vi "Build BC Schedule.vi"(8 "error in (no error)":errorcluster, 11 "Bus Controller in":refnum<class "Bus Controller.lvclass">) -> (0 "error out":errorcluster, 3 "Bus Controller out":refnum<class "Bus Controller.lvclass">)   [LabVIEW 2020, in "Unit Tests.lvlib" / "Bus Controller.lvclass"]
uses:
  Bus Controller.lvclass
  Bus Controller/TypeDefs/Bus Controller Configuration.ctl
  Bus Controller/TypeDefs/Bus Controller Timeout.ctl
  Frames & Messages/TypeDefs/RT-RT Message Config.ctl
  Frames & Messages/TypeDefs/Command Config.ctl
  Frames & Messages/TypeDefs/Command Type.ctl
  Frames & Messages/TypeDefs/Command Terminal Address.ctl
  Frames & Messages/TypeDefs/Command SubAddress.ctl
  Frames & Messages/TypeDefs/Command Word Count.ctl
  Frames & Messages/TypeDefs/Message Config.ctl
  Frames & Messages/TypeDefs/Message Control.ctl
  Frames & Messages/TypeDefs/Simplified Parameter Data Table.ctl
  Frames & Messages/TypeDefs/Scaling Information.ctl
  Bus Controller.lvclass/Bus Controller.ctl
  Frames & Messages/RT-RT Message/RT-RT Message.lvclass
  C:/Users/MattJ/Desktop/git/bci-1553-labview-api/src/Frames & Messages/Message/Message.lvclass
  Bus Controller/Bus Controller.lvclass
  C:/Users/MattJ/Desktop/git/bci-1553-labview-api/src/1553 SubComponent/1553 SubComponent.lvclass
  Frames & Messages/Major Frame/Major Frame.lvclass
  1553 Session/1553 Session.lvclass
  BCI-1553 API.lvlib
  Frames & Messages/Message/Message.lvclass
  Frames & Messages/Minor Frame/Minor Frame.lvclass
  1553 Component/1553 Component.lvclass
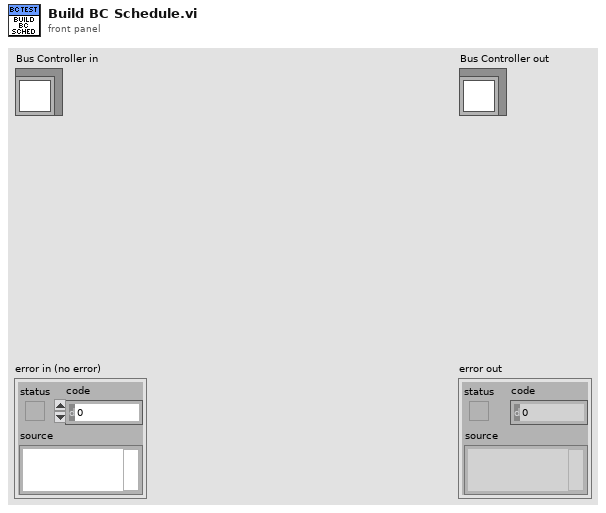
[diagram p1: front panel]
types:
  T1 = typedef "BCI-1553 API.lvlib/Command Type.ctl" = enum16{"Transmit", "Receive"}
  T2 = typedef "BCI-1553 API.lvlib/Command Terminal Address.ctl" = enum16{"0", "1", "2", "3", "4", "5", "6", "7", "8", "9", "10", "11", "12", "13", "14", "15", "16", "17", "18", "19", "20", "21", "22", "23", "24", "25", "26", "27", "28", "29", "30", "Broadcast"}
  T3 = typedef "BCI-1553 API.lvlib/Command SubAddress.ctl" = enum16{"Mode Code", "1", "2", "3", "4", "5", "6", "7", "8", "9", "10", "11", "12", "13", "14", "15", "16", "17", "18", "19", "20", "21", "22", "23", "24", "25", "26", "27", "28", "29", "30"}
  T4 = typedef "BCI-1553 API.lvlib/Command Word Count.ctl" = enum16{"1", "2", "3", "4", "5", "6", "7", "8", "9", "10", "11", "12", "13", "14", "15", "16", "17", "18", "19", "20", "21", "22", "23", "24", "25", "26", "27", "28", "29", "30", "31", "32"}
  T5 = typedef "BCI-1553 API.lvlib/Message Config.ctl" = cluster{"Time to Next Msg (4 us)":u16, "Command Config":T6, "Message Control":T7}
  T6 = typedef "BCI-1553 API.lvlib/Command Config.ctl" = cluster{"Command Type":T1, "Terminal Address":T2, "SubAddress":T3, "Word Count\\Mode Code":T4, "Command Data":u16[]}
  T7 = typedef "BCI-1553 API.lvlib/Message Control.ctl" = cluster{"MC17 Time Sync":bool, "Error Mask":bool, "Service Request Mask":bool, "Busy Mask":bool, "SubSystem Flag Mask":bool, "Terminal Flag Mask":bool, "Reserved Mask":bool, "Retry":bool, "Bus A / !Bus B":bool, "Self-Test Loopback":bool, "Broadcast Mask":bool, "EoM Interrupt":bool, "Mode Code Format":bool, "Broadcast Format":bool, "RT-RT Format":bool}
  T8 = typedef "BCI-1553 API.lvlib/RT-RT Message Config.ctl" = cluster{"Tx Command Config":T6}
  T9 = typedef "BCI-1553 API.lvlib/Bus Controller.lvclass/Bus Controller Configuration.ctl" = cluster{"Timeout":T10, "BC Retry":bool, "BC Second Retry":bool, "BC Retry Alt Bus":bool, "BC Second Retry Alt Bus":bool, "BC Retry on Status Bit":bool, "Msg Error No Data Valid":bool, "Busy Status No Data Valid":bool, "Msg Gap Timer":bool, "Watchdog Timer":bool, "Time Tag Sync":bool, "Even Time Tag Sync":bool, "Gap Check":bool, "Broadcast Mask Enable":bool}
  T10 = typedef "BCI-1553 API.lvlib/Bus Controller.lvclass/Bus Controller Timeout.ctl" = enum16{"17us", "22us", "60us", "140us"}
  T11 = typedef "BCI-1553 API.lvlib/Simplified Parameter Data Table.ctl" = cluster{"Parameter Name":string, "Base Word":u16, "Scaling Info":T12}
  T12 = typedef "BCI-1553 API.lvlib/Scaling Information.ctl" = cluster{"Bit Offset":i32, "Bit Count":i32, "LSB Resolution":dbl, "2's Complement":bool, "Big Endian":bool, "Sign Bit":bool}
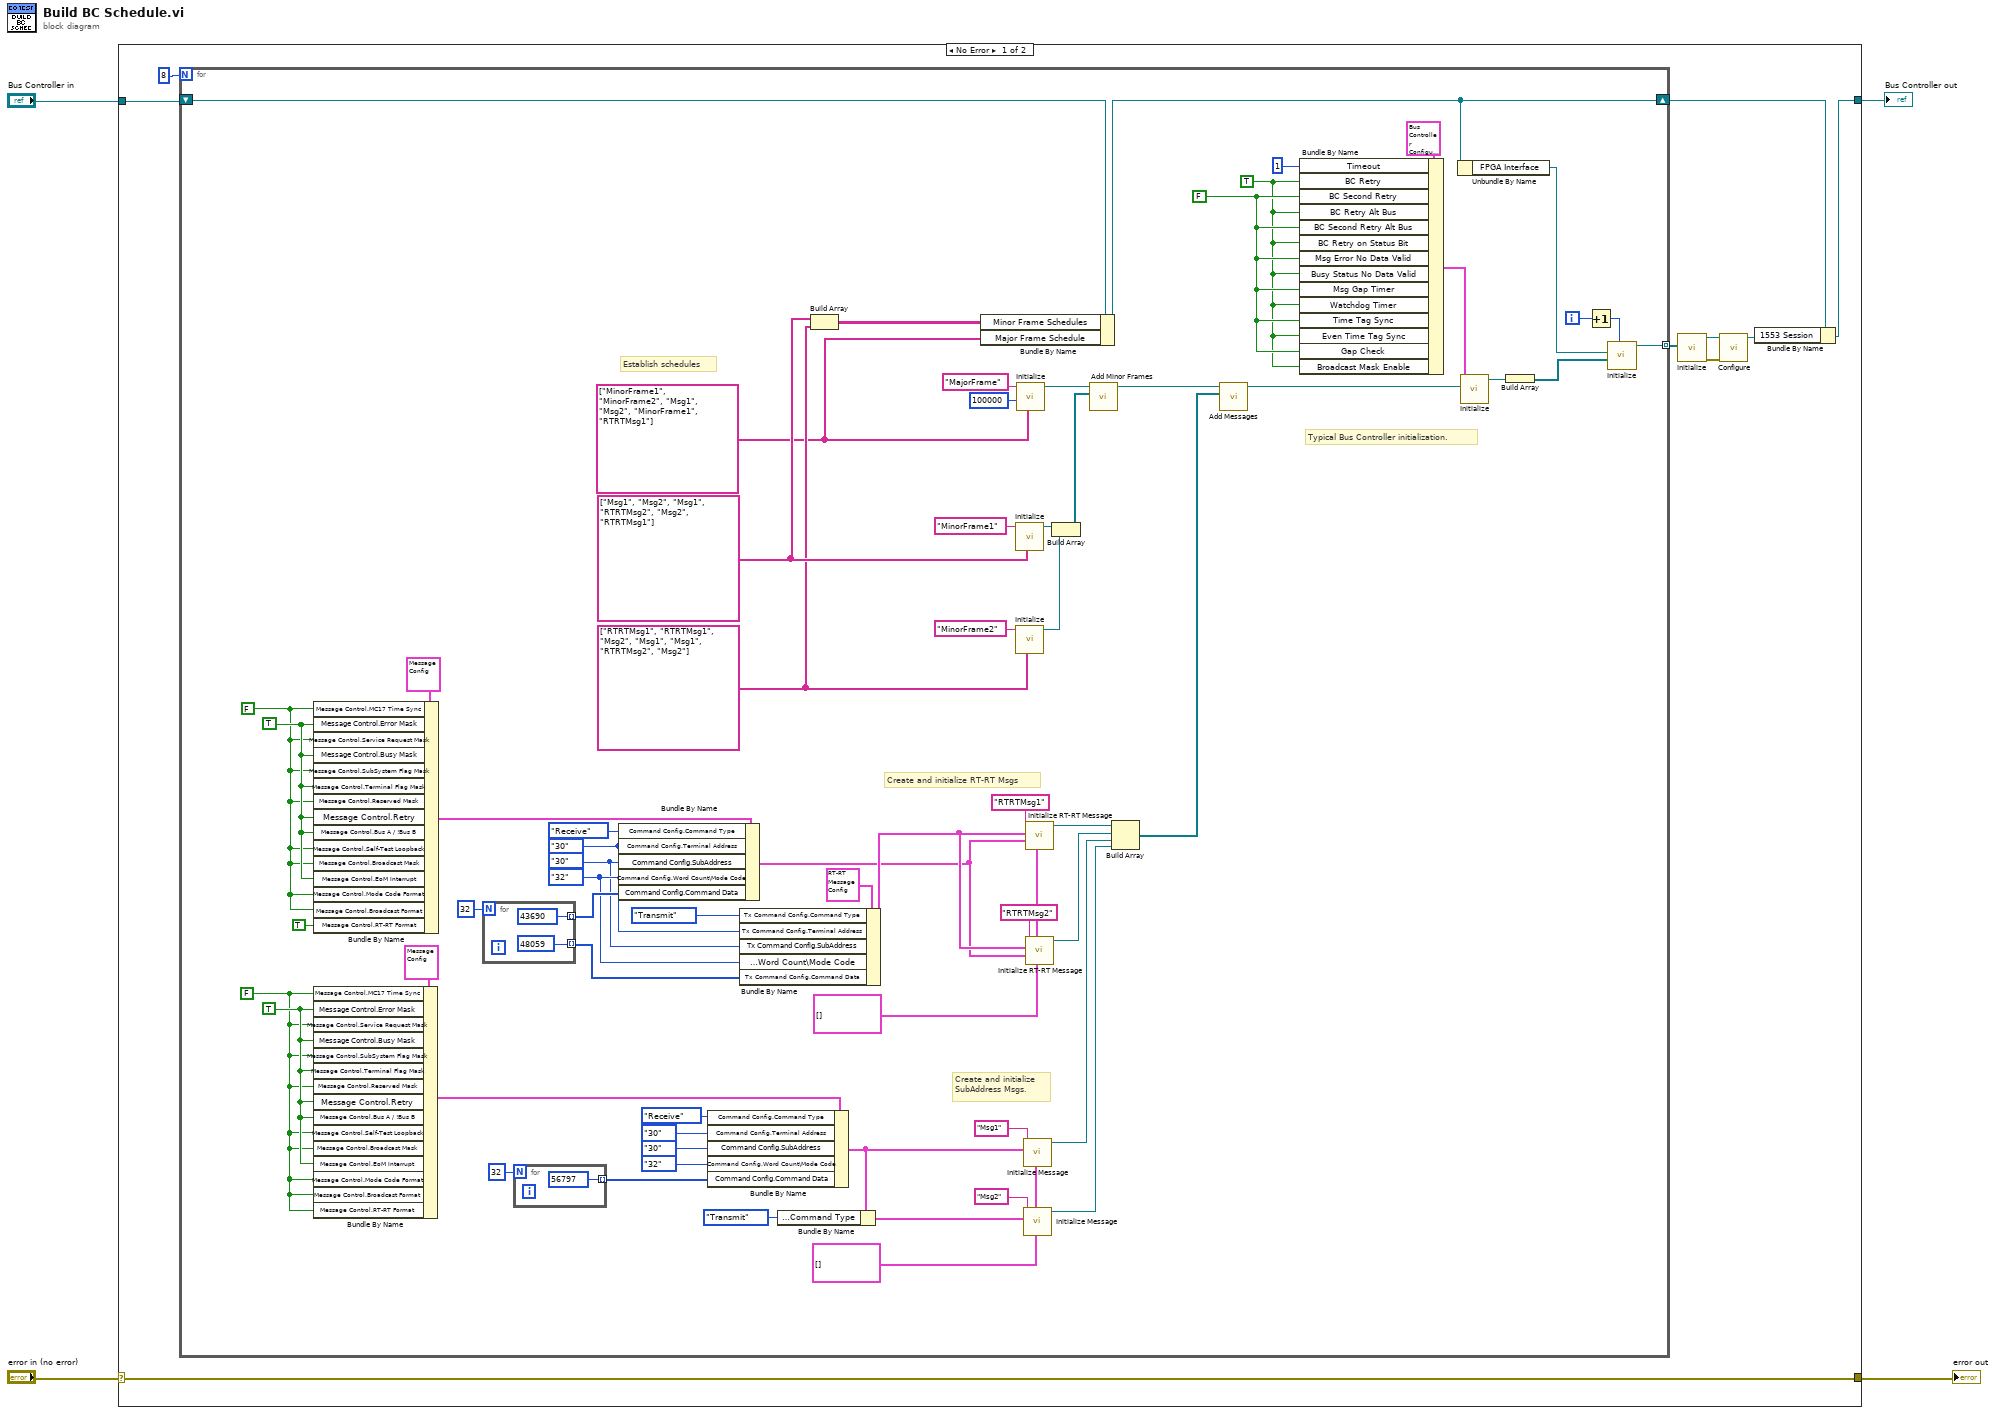
[diagram p0: block diagram]
diagram:
  n1 = case shown="No Error" "error in (no error)" {
    selector: "error in (no error)" -> [w8 w85]
    tunnel: [w8 w85] -> w3
    tunnel: [w6 w84] -> w1
    tunnel: "Bus Controller in" -> [w12 w84]
    frame No Error {
      n2 = for {
        N: 8 -> [_]
        shift-right: [w23] -> w7
        shift-left: w12 -> [w46]
        tunnel: [w39] -> w11 mode=indexing
        i -> [w38]
        w27 = string[] ["Msg1", "Msg2", "Msg1", "RTRTMsg2", "Msg2", "RTRTMsg1"]
        w25 = string[] ["RTRTMsg1", "RTRTMsg1", "Msg2", "Msg1", "Msg1", "RTRTMsg2", "Msg2"]
        w24 = string[] ["MinorFrame1", "MinorFrame2", "Msg1", "Msg2", "MinorFrame1", "RTRTMsg1"]
        w20 = T11[] [] ("Parameters")
        w21 = T11[] [] ("Parameters")
        w30 = Command_Terminal_Address."30" ("Command Config.Terminal Address")
        w31 = Command_SubAddress."30" ("Command Config.SubAddress")
        w32 = Command_Word_Count."32" ("Command Config.Word Count\\Mode Code")
        w52 = TRUE ("Message Control.Error Mask")
        w51 = FALSE ("Message Control.MC17 Time Sync")
        w57 = TRUE ("Message Control.Error Mask")
        w55 = FALSE ("Message Control.MC17 Time Sync")
        w74 = FALSE ("BC Second Retry")
        w73 = TRUE ("BC Retry")
        # "Create and initialize RT-RT Msgs"
        # "Establish schedules"
        # "Create and initialize\nSubAddress Msgs."
        # "Typical Bus Controller initialization."
        n3 = Bundle By Name(cluster=T5 {"Time to Next Msg (4 us)"=100, "Command Config"={"Command Type"=enum."Transmit", "Terminal Address"=enum."0", "SubAddress"=enum."Mode Code", "Word Count\\Mode Code"=enum."1", "Command Data"=[]}, "Message Control"={"MC17 Time Sync"=FALSE, "Error Mask"=FALSE, "Service Request Mask"=FALSE, "Busy Mask"=FALSE, "SubSystem Flag Mask"=FALSE, "Terminal Flag Mask"=FALSE, "Reserved Mask"=FALSE, "Retry"=FALSE, "Bus A / !Bus B"=FALSE, "Self-Test Loopback"=FALSE, "Broadcast Mask"=FALSE, "EoM Interrupt"=FALSE, "Mode Code Format"=FALSE, "Broadcast Format"=FALSE, "RT-RT Format"=FALSE}} ("Message Config"), "Message Control.MC17 Time Sync"=w51, "Message Control.Error Mask"=w52, "Message Control.Service Request Mask"=w51, "Message Control.Busy Mask"=w52, "Message Control.SubSystem Flag Mask"=w51, "Message Control.Terminal Flag Mask"=w52, "Message Control.Reserved Mask"=w51, "Message Control.Retry"=w52, "Message Control.Bus A / !Bus B"=w52, "Message Control.Self-Test Loopback"=w51, "Message Control.Broadcast Mask"=w51, "Message Control.EoM Interrupt"=w52, "Message Control.Mode Code Format"=w51, "Message Control.Broadcast Format"=w51, "Message Control.RT-RT Format"=w51) -> (w18:T5)
        n4 = Bundle By Name(cluster=T5 {"Time to Next Msg (4 us)"=100, "Command Config"={"Command Type"=enum."Transmit", "Terminal Address"=enum."0", "SubAddress"=enum."Mode Code", "Word Count\\Mode Code"=enum."1", "Command Data"=[]}, "Message Control"={"MC17 Time Sync"=FALSE, "Error Mask"=FALSE, "Service Request Mask"=FALSE, "Busy Mask"=FALSE, "SubSystem Flag Mask"=FALSE, "Terminal Flag Mask"=FALSE, "Reserved Mask"=FALSE, "Retry"=FALSE, "Bus A / !Bus B"=FALSE, "Self-Test Loopback"=FALSE, "Broadcast Mask"=FALSE, "EoM Interrupt"=FALSE, "Mode Code Format"=FALSE, "Broadcast Format"=FALSE, "RT-RT Format"=FALSE}} ("Message Config"), "Message Control.MC17 Time Sync"=w55, "Message Control.Error Mask"=w57, "Message Control.Service Request Mask"=w55, "Message Control.Busy Mask"=w57, "Message Control.SubSystem Flag Mask"=w55, "Message Control.Terminal Flag Mask"=w57, "Message Control.Reserved Mask"=w55, "Message Control.Retry"=w57, "Message Control.Bus A / !Bus B"=w57, "Message Control.Self-Test Loopback"=w55, "Message Control.Broadcast Mask"=w55, "Message Control.EoM Interrupt"=w57, "Message Control.Mode Code Format"=w55, "Message Control.Broadcast Format"=w55, "Message Control.RT-RT Format"=TRUE) -> (w19:T5)
        n5 = for {
          N: 32 -> [_]
          tunnel: [u16 43690] -> w44 mode=indexing
          tunnel: [u16 48059] -> w43 mode=indexing
        }
        n6 = for {
          N: 32 -> [_]
          tunnel: [u16 56797] -> w49 mode=indexing
        }
        n7 = Bundle By Name(cluster=w19, "Command Config.Command Type"=Command_Type."Receive", "Command Config.Terminal Address"=w30, "Command Config.SubAddress"=w31, "Command Config.Word Count\\Mode Code"=w32, "Command Config.Command Data"=w44) -> (w41:T5)
        n8 = Bundle By Name(cluster=w18, "Command Config.Command Type"=Command_Type."Receive", "Command Config.Terminal Address"=Command_Terminal_Address."30", "Command Config.SubAddress"=Command_SubAddress."30", "Command Config.Word Count\\Mode Code"=Command_Word_Count."32" ("Command Config.Word Count\\Mode Code"), "Command Config.Command Data"=w49) -> (w48:T5)
        n9 = Bundle By Name(cluster=T8 {"Tx Command Config"={"Command Type"=enum."Transmit", "Terminal Address"=enum."0", "SubAddress"=enum."Mode Code", "Word Count\\Mode Code"=enum."1", "Command Data"=[]}} ("RT-RT Message Config"), "Tx Command Config.Command Type"=Command_Type."Transmit", "Tx Command Config.Terminal Address"=w30, "Tx Command Config.SubAddress"=w31, "Tx Command Config.Word Count\\Mode Code"=w32, "Tx Command Config.Command Data"=w43) -> (w42:T8)
        n10 = Bundle By Name(cluster=w48, "Command Config.Command Type"=Command_Type."Transmit") -> (w47:T5)
        n11 = Build Array(w27, w25) -> (w45:string[][])
        n12 = Bundle By Name(cluster=w46, "Minor Frame Schedules"=w45, "Major Frame Schedule"=w24) -> (w23:refnum<class "Bus Controller.lvclass">)
        n13 = call "Initialize.vi"("Schedule"=w27, "ID"="MinorFrame1") -> ("Minor Frame out"=w70:refnum<class "Minor Frame.lvclass">)  [unwired: 8 in, 1 out]
        n14 = call "Initialize.vi"("Schedule"=w25, "ID"="MinorFrame2") -> ("Minor Frame out"=w69:refnum<class "Minor Frame.lvclass">)  [unwired: 8 in, 1 out]
        n15 = call "Initialize.vi"("Schedule"=w24, "Minor Frame Time (100 us)"=u32 100000, "ID"="MajorFrame") -> ("Major Frame out"=w72:refnum<class "Major Frame.lvclass">)  [unwired: 7 in, 1 out]
        n16 = call "Initialize Message.vi"("Parameters"=w21, "Message  Config"=w48, "ID"="Msg1") -> ("Message out"=w61:refnum<class "Message.lvclass">)  [unwired: 7 in, 1 out]
        n17 = call "Initialize Message.vi"("Parameters"=w21, "Message  Config"=w47, "ID"="Msg2") -> ("Message out"=w64:refnum<class "Message.lvclass">)  [unwired: 7 in, 1 out]
        n18 = call "Initialize RT-RT Message.vi"("Parameters"=w20, "Receive Message Config"=w41, "Transmit Message Config"=w42, "ID"="RTRTMsg1") -> ("RT-RT Message out"=w65:refnum<class "RT-RT Message.lvclass">)  [unwired: 6 in, 1 out]
        n19 = call "Initialize RT-RT Message.vi"("Parameters"=w20, "Receive Message Config"=w41, "Transmit Message Config"=w42, "ID"="RTRTMsg2") -> ("RT-RT Message out"=w60:refnum<class "RT-RT Message.lvclass">)  [unwired: 6 in, 1 out]
        n20 = Build Array(w70, w69) -> (w68:refnum<class "Minor Frame.lvclass">[])
        n21 = call-dynamic "Add Minor Frames.vi"("Minor Frames"=w68, "Major Frame in"=w72) -> ("Major Frame out"=w67:refnum<class "Major Frame.lvclass">)  [unwired: 8 in, 1 out]
        n22 = Build Array(w65, w60, w61, w64) -> (w63:refnum<class "Message.lvclass">[])
        n23 = call-dynamic "Add Messages.vi"("Messages"=w63, "Major Frame in"=w67) -> ("Major Frame out"=w62:refnum<class "Major Frame.lvclass">)  [unwired: 8 in, 1 out]
        n24 = Bundle By Name(cluster=T9 {"Timeout"=enum."17us", "BC Retry"=FALSE, "BC Second Retry"=FALSE, "BC Retry Alt Bus"=FALSE, "BC Second Retry Alt Bus"=FALSE, "BC Retry on Status Bit"=FALSE, "Msg Error No Data Valid"=FALSE, "Busy Status No Data Valid"=FALSE, "Msg Gap Timer"=FALSE, "Watchdog Timer"=FALSE, "Time Tag Sync"=FALSE, "Even Time Tag Sync"=FALSE, "Gap Check"=FALSE, "Broadcast Mask Enable"=FALSE} ("Configuration"), "Timeout"=u16 1 ("BC Timeout"), "BC Retry"=w73, "BC Second Retry"=w74, "BC Retry Alt Bus"=w73, "BC Second Retry Alt Bus"=w74, "BC Retry on Status Bit"=w73, "Msg Error No Data Valid"=w74, "Busy Status No Data Valid"=w73, "Msg Gap Timer"=w74, "Watchdog Timer"=w73, "Time Tag Sync"=w74, "Even Time Tag Sync"=w73, "Gap Check"=w74, "Broadcast Mask Enable"=w73) -> (w76:T9)
        n25 = Unbundle By Name(w23) -> ("FPGA Interface"=w22:refnum<class "FPGA Interface.lvclass">)
        n26 = call "Initialize.vi"("Major Frame"=w62, "Configuration"=w76) -> ("Bus Controller out"=w79:refnum<class "Bus Controller.lvclass">)  [unwired: 8 in, 1 out]
        n27 = Build Array(w79) -> (w78:refnum<class "Bus Controller.lvclass">[])
        n28 = Increment(x=w38) -> (x+1=w40:i32)
        n29 = call "Initialize.vi"("Component ID (1-8)"=w40, "SubComponents"=w78, "FPGA Interface"=w22) -> ("1553 Component out"=w39:refnum<class "1553 Component.lvclass">)  [unwired: 7 in, 1 out]
      }
      n30 = call "Initialize.vi"("Components"=w11) -> ("error out"=w9:errorcluster, "1553 Board out"=w10:refnum<class "1553 Session.lvclass">)  [unwired: 9 in]
      n31 = call-dynamic "Configure.vi"("error in (no error)"=w9, "1553 Board in"=w10) -> ("1553 Board out"=w5:refnum<class "1553 Session.lvclass">)  [unwired: 8 in, 1 out]
      n32 = Bundle By Name(cluster=w7, "1553 Session"=w5) -> (w6:refnum<class "Bus Controller.lvclass">)
    }
    frame Error {
    }
  }
  "error out" <- w3
  "Bus Controller out" <- w1
